vi "WPI_ADI_IMU_Close.vi"(8 "error in":errorcluster, 11 "ADI IMU DevRef":T1 {"Sample Rate" min=0.25 max=100.0 step=0.25}) -> (0 "error out":errorcluster)   [LabVIEW 2015, in "FRC ADI MXP IMU.lvlib"]
doc: "Closes the ADIIMUDevRef and properly shuts down SPI communication between the RoboRIO and the ADI IMU MXP board."
uses:
  FRC ADI MXP IMU.lvlib
  WPI_AnalogDevicesIMUDevRef.ctl
  <vilib>/Rock Robotics/SystemInterfaces/spilib/spi_bus.ctl
  <vilib>/Rock Robotics/WPI/SPI/WPI_SPIDevRef.ctl
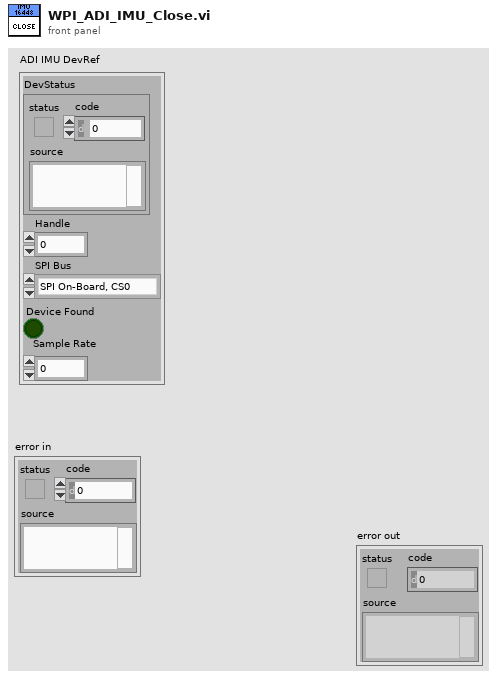
[diagram p1: front panel]
types:
  T1 = typedef "FRC ADI MXP IMU.lvlib/WPI_AnalogDevicesIMUDevRef.ctl" = cluster{"DevStatus":errorcluster, "Handle":i32, "SPI Bus":T2, "Device Found":bool, "Sample Rate":dbl}
  T2 = typedef "spi_bus.ctl" = enum16{"SPI On-Board, CS0", "SPI On-Board, CS1", "SPI On-Board, CS2", "SPI On-Board, CS3", "SPI MXP", "Invalid"}
  T3 = typedef "WPI_SPIDevRef.ctl" = cluster{"DevStatus":errorcluster, "Handle":i32, "SPI Bus":T2}
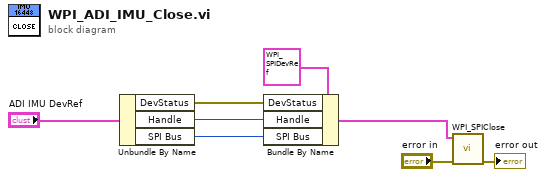
[diagram p0: block diagram]
diagram:
  n1 = Unbundle By Name("ADI IMU DevRef") -> ("DevStatus"=w4:errorcluster, "Handle"=w3:i32, "SPI Bus"=w2:T2)
  n2 = Bundle By Name(cluster=T3 {"DevStatus"={"status"=FALSE, "code"=0, "source"=""}, "Handle"=0, "SPI Bus"=enum."SPI On-Board, CS0"} ("SPIDevRef"), "DevStatus"=w4, "Handle"=w3, "SPI Bus"=w2) -> (w1:T3)
  n3 = call <vilib>:"WPI_SPIClose.vi"("error in (no error)"="error in", "SPIDevRef"=w1) -> ("error out"=→"error out":errorcluster)  [unwired: 9 in]
